vi "Write State.vi"(8 "error in (no error)":errorcluster, 10 "State":T1, 11 "Expansion in":refnum<class "Recipes.lvclass">) -> (0 "error out":errorcluster, 3 "Expansion out":refnum<class "Recipes.lvclass">)   [LabVIEW 2017, in "Recipes.lvclass"]
uses:
  Recipes.lvclass
  Type Defs/Recipes State.ctl
  Recipes.lvclass/Recipes.ctl
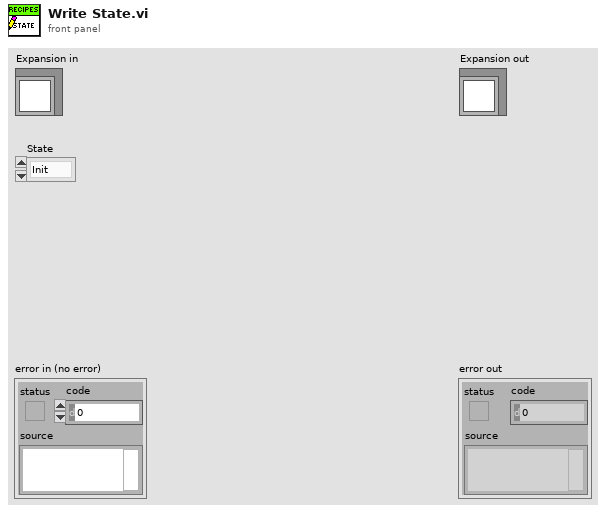
[diagram p1: front panel]
types:
  T1 = typedef "Recipes.lvclass/Recipes State.ctl" = enum16{"Init", "Go", "Stop", "Idle", "Error", "Shutdown"}
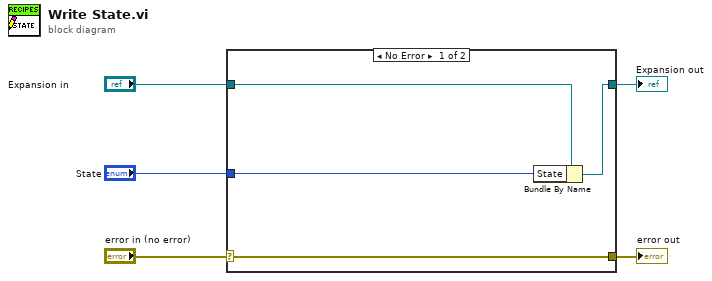
[diagram p0: block diagram]
diagram:
  n1 = case shown="No Error" "error in (no error)" {
    selector: "error in (no error)" -> [w9 w10]
    tunnel: [w9 w10] -> w4
    tunnel: [w7 w11] -> w2
    tunnel: "Expansion in" -> [w8 w11]
    tunnel: "State" -> [w6 _]
    frame No Error {
      n2 = Bundle By Name(cluster=w8, "State"=w6) -> (w7:refnum<class "Recipes.lvclass">)
    }
    frame Error {
    }
  }
  "error out" <- w4
  "Expansion out" <- w2
